vi "Python_Calibration.vi"() -> (0 "error out 2":errorcluster)   [LabVIEW 2021]
doc: "This example demonstrates how to call a Python function and pass integers as arguments. It uses a python function to compute the sum of two integers."
uses:
  Global_Variables.vi
panel:
  in  "error in (no error) 2":errorcluster
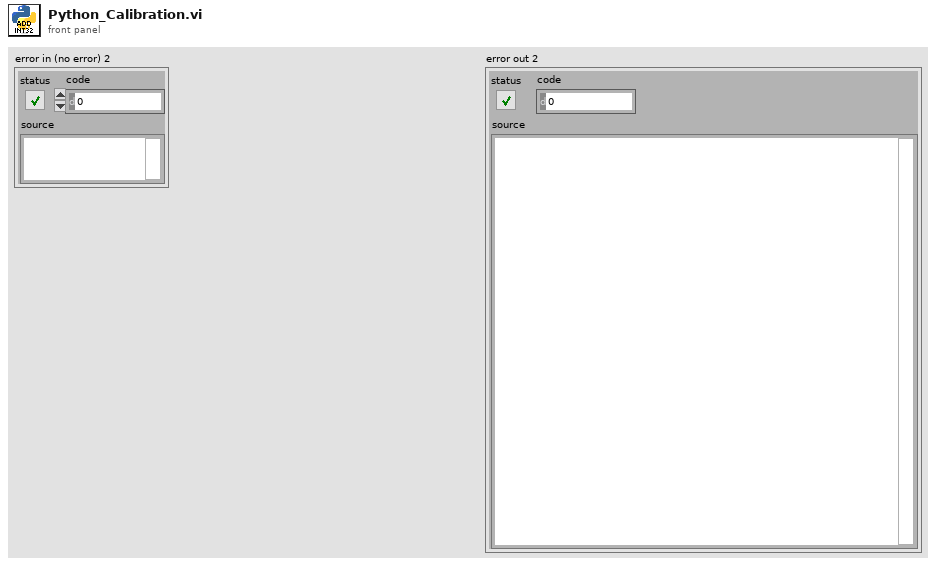
[diagram p1: front panel]
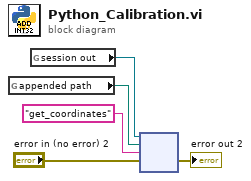
[diagram p0: block diagram]
diagram:
  n1 = global read "Global_Variables.vi" "appended path"() -> (w2:path)
  n2 = global read "Global_Variables.vi" "session out"() -> (w1:refnum<k35>)
  n3 = node(w1, w2, "get_coordinates" ("function name"), "error in (no error) 2") -> (→"error out 2":errorcluster)  [unwired: 2 in, 3 out]
